vi "AGCxxx Transaction.vi"(7 "error in (no error)":errorcluster, 8 "Bytes to read (100)":u32=100, 9 "AGC Command String":string, 10 "AGCxxx VISA Cluster":T1={"VISA resource name"="", "VISA Timeout Value (1000 ms)"=1000, "Lock Timeout (1000 ms)"=1000, "MAX Channel (6)"=6}) -> (0 "error out":errorcluster, 1 "AGC Errno":i32, 2 "AGC Response":string, 3 "dup AGCxxx VISA Cluster":T1={"VISA resource name"="", "VISA Timeout Value (1000 ms)"=1000, "Lock Timeout (1000 ms)"=1000, "MAX Channel (6)"=6})   [LabVIEW 2014, in "AGCxxx - Driver.lvlib"]
doc: "Makes the transaction with the AGC,\nformating command or query strings, \nsends and reads strings\nlocks and unlocks the VISA source\n\n \n\nCopyright (C) \nGesellschaft f. Schwerionenforschung, GSI\nPlanckstr. 1\n64291 Darmstadt\nGermany\n\nContact: http://www-wnt.gsi.de/labview\n H.Brand@gsi.de\n\nThis program is free software; you can redistribute it and/or\nmodify it under the terms of the GNU General Public License\nas published by the Free Software Foundation; either version 2\nof the License, or (at your option) any later version.\n\nThis program is distributed in the hope that it will be useful,\nbut WITHOUT ANY WARRANTY; without even the implied warranty of\nMERCHANTABILITY or FITNESS FOR A PARTICULAR PURPOSE. See the\nGNU General Public License for more details (http://www.gnu.org)."
uses:
  AGCxxx - Driver.lvlib
  AGCxxx VISA Control.ctl
panel:
  out "write buffer (\"\")":string
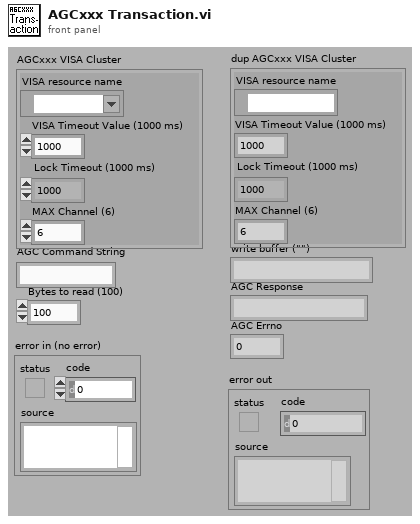
[diagram p1: front panel]
types:
  T1 = typedef "AGCxxx - Driver.lvlib/AGCxxx VISA Control.ctl" = cluster{"VISA resource name":refnum<visa-resource-name>, "VISA Timeout Value (1000 ms)":u32, "Lock Timeout (1000 ms)":u32, "MAX Channel (6)":i32}
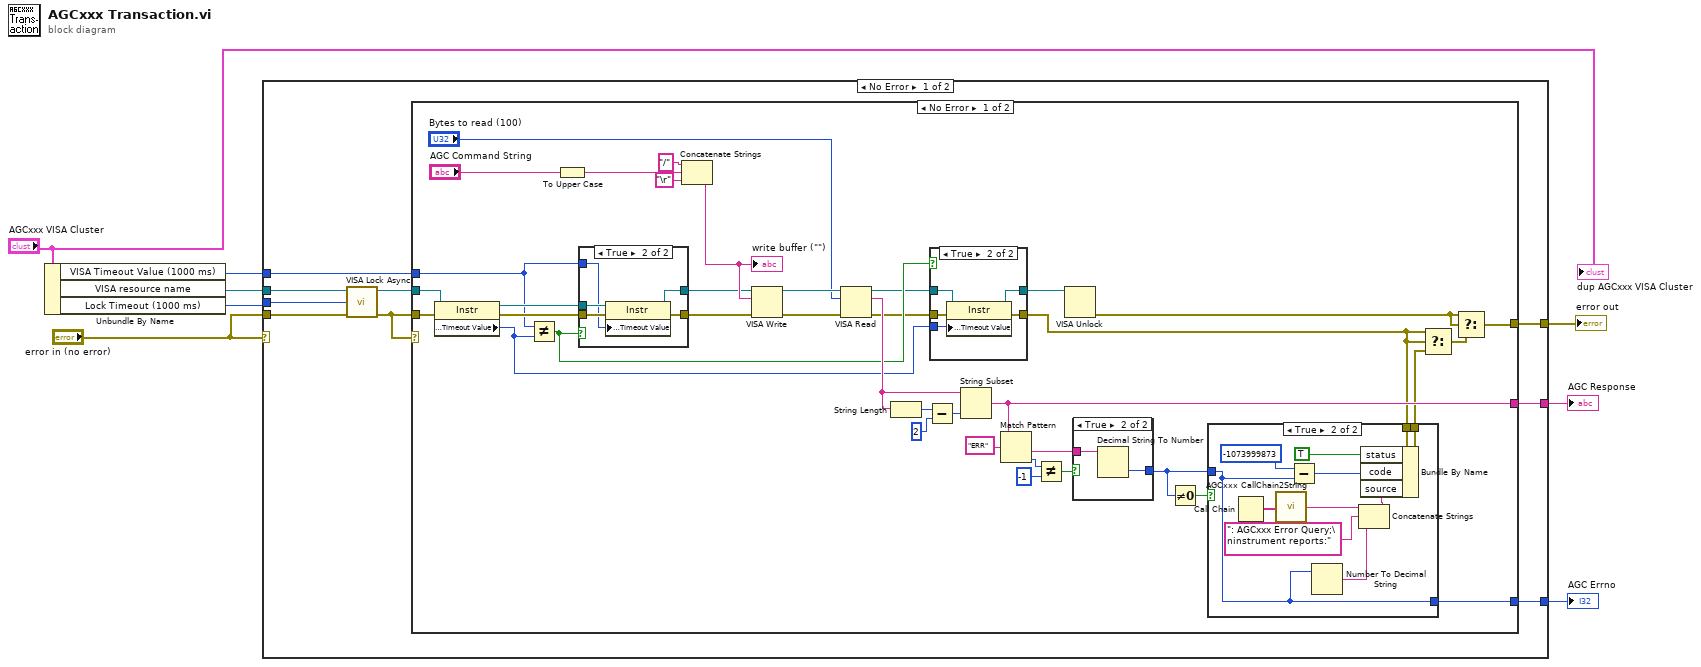
[diagram p0: block diagram]
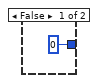
[diagram p3: hidden frame]
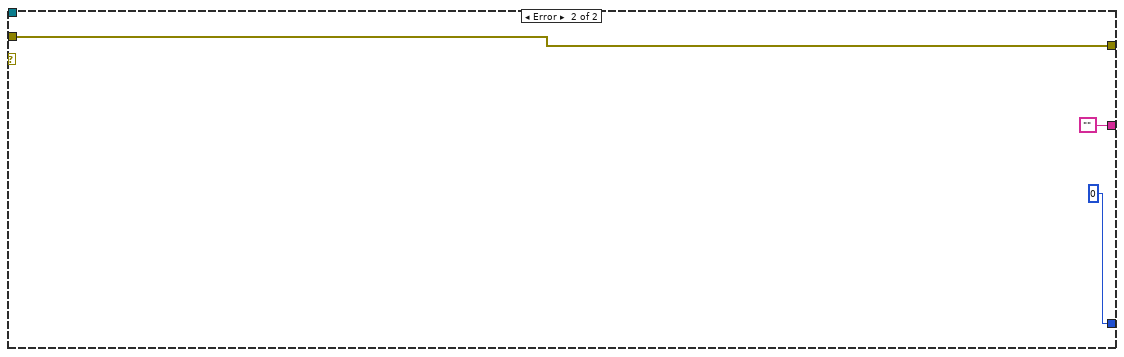
[diagram p6: hidden frame]
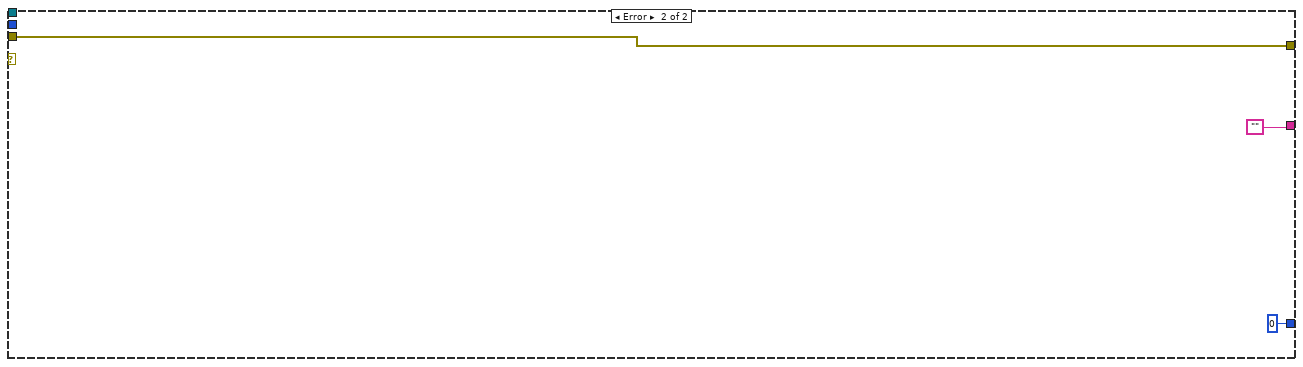
[diagram p7: hidden frame]
diagram:
  n1 = Unbundle By Name("AGCxxx VISA Cluster") -> ("VISA Timeout Value (1000 ms)"=w3:u32, "VISA resource name"=w1:refnum<visa-resource-name>, "Lock Timeout (1000 ms)"=w2:u32)
  n2 = case shown="No Error" "error in (no error)" {
    tunnel: w1 -> [w16 _]
    tunnel: "error in (no error)" -> [w15 w91]
    tunnel: [w13 ""] -> w7
    tunnel: [w12 w91] -> w5
    tunnel: [w11 0] -> w8
    tunnel: w2 -> [w10 _]
    tunnel: w3 -> [w9 _]
    frame No Error {
      n3 = call <vilib>:"VISA Lock Async.vi"("error in (no error)"=w15, "timeout (0)"=w10, "VISA resource name"=w16) -> ("error out"=w14:errorcluster, "VISA resource name out"=w17:refnum<visa-resource-name>)  [unwired: 6 in, 1 out]
      n4 = case shown="No Error" w14 {
        tunnel: w17 -> [w44 _]
        tunnel: w14 -> [w41 w88]
        tunnel: [w36 "" ("read buffer")] -> w13
        tunnel: [w21 w88] -> w12
        tunnel: [w25 0] -> w11
        tunnel: w9 -> [w23 _]
        frame No Error {
          n5 = property class="Instr"(reference=w44, error in=w41) -> (reference out=w43:refnum<visa-resource-name>, error out=w40:errorcluster, "General Settings:Timeout Value"=w38:u32)
          n6 = Not Equal?(x=w23, y=w38) -> (x != y?=w37:bool)
          n7 = To Upper Case(1:"AGC Command String") -> (0:w24:string)
          n8 = case shown="True" w37 {
            tunnel: w43 -> [w80 w85]
            tunnel: [w80 w84] -> w42
            tunnel: w40 -> [w79 w83]
            tunnel: [w79 w82] -> w39
            tunnel: w23 -> [_ w81]
            frame False {
            }
            frame True {
              n9 = property class="Instr"(reference=w85, error in=w83, "General Settings:Timeout Value"=w81) -> (reference out=w84:refnum<visa-resource-name>, error out=w82:errorcluster)
            }
          }
          n10 = Concatenate Strings("/" ("Substring"), w24, "\r" ("Substring")) -> (w52:string)
          "write buffer (\"\")" <- w52
          n11 = VISA Write(VISA resource name=w42, write buffer=w52, error in (no error)=w39) -> (VISA resource name out=w54:refnum<visa-resource-name>, error out=w55:errorcluster)  [unwired: 1 out]
          n12 = VISA Read(VISA resource name=w54, byte count="Bytes to read (100)", error in (no error)=w55) -> (VISA resource name out=w30:refnum<visa-resource-name>, read buffer=w48:string, error out=w29:errorcluster)  [unwired: 1 out]
          n13 = String Length(string=w48) -> (length=w47:i32)
          n14 = Subtract(x=w47, y=2) -> (x-y=w45:i32)
          n15 = case shown="True" w37 {
            tunnel: w30 -> [w73 w78]
            tunnel: [w73 w77] -> w28
            tunnel: w29 -> [w72 w76]
            tunnel: [w72 w75] -> w20
            tunnel: w38 -> [_ w74]
            frame False {
            }
            frame True {
              n16 = property class="Instr"(reference=w78, error in=w76, "General Settings:Timeout Value"=w74) -> (reference out=w77:refnum<visa-resource-name>, error out=w75:errorcluster)
            }
          }
          n17 = String Subset(string=w48, length (rest)=w45) -> (substring=w36:string)  [unwired: 1 in]
          n18 = Match Pattern(string=w36, regular expression="ERR") -> (after substring=w31:string, offset past match=w34:i32)  [unwired: 1 in, 2 out]
          n19 = Not Equal?(x=w34, y=-1) -> (x != y?=w32:bool)
          n20 = VISA Unlock(11:w28) -> (0:w22:errorcluster)  [unwired: 1 in, 1 out]
          n21 = case shown="True" w32 {
            tunnel: w31 -> [_ w71]
            tunnel: [0 w70] -> w27
            frame False {
            }
            frame True {
              n22 = Decimal String To Number(string=w71) -> (number=w70:i32)  [unwired: 2 in, 1 out]
            }
          }
          n23 = Not Equal To 0?(x=w27) -> (x != 0?=w26:bool)
          n24 = case shown="True" w26 {
            tunnel: w27 -> [w56 w59]
            tunnel: [w57 w67] -> w18
            tunnel: w20 -> [w57 w66]
            tunnel: [w56 w59] -> w25
            frame False {
            }
            frame True {
              n25 = Call Chain() -> (call chain=w63:string[])
              n26 = call "AGCxxx CallChain2String.vi"("call chain"=w63) -> ("Call Chain String"=w61:string)
              n27 = Subtract(x=-1073999873, y=w59) -> (x-y=w64:i32)
              n28 = Number To Decimal String(number=w59) -> (decimal integer string=w58:string)  [unwired: 1 in]
              n29 = Concatenate Strings(w61, ": AGCxxx Error Query;\ninstrument reports:", w58) -> (w62:string)
              n30 = Bundle By Name(cluster=w66, "status"=TRUE, "code"=w64, "source"=w62) -> (w67:errorcluster)
            }
          }
          n31 = Select(t=w20, s=w20, f=w18) -> (s? t:f=w19:errorcluster)
          n32 = Select(t=w22, s=w22, f=w19) -> (s? t:f=w21:errorcluster)
        }
        frame Error {
        }
      }
    }
    frame Error {
    }
  }
  "AGC Errno" <- w8
  "AGC Response" <- w7
  "error out" <- w5
  "dup AGCxxx VISA Cluster" <- "AGCxxx VISA Cluster"
